vi "UE9 Pin Configuration.vi"(4 "Enable Counter1":bool, 6 "Enable Counter0":bool, 8 "error in":errorcluster, 9 "Enable DACs":bool, 10 "Number of Timers Enabled":u8, 11 "Handle In":i32) -> (0 "error out":errorcluster, 3 "Handle Out":i32)   [LabVIEW 2021]
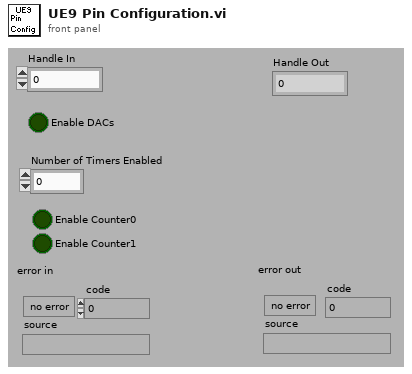
[diagram p1: front panel]
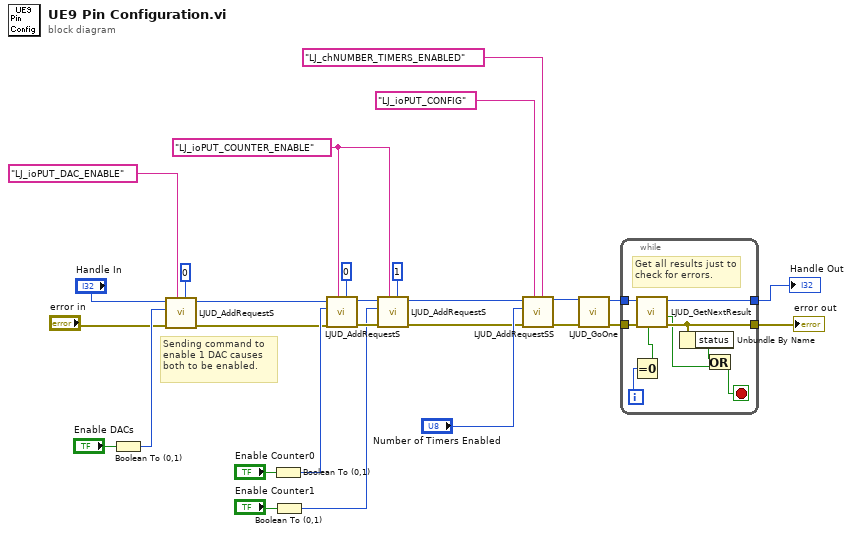
[diagram p0: block diagram]
diagram:
  w19 = "LJ_ioPUT_COUNTER_ENABLE" ("Channel")
  # "Sending command to\nenable 1 DAC causes\nboth to be enabled."
  n1 = Boolean To (0,1)(Boolean="Enable DACs") -> (0, 1=w5:i16)
  n2 = call "LJUD_AddRequestS.vi"("Channel"=0, "IOType"="LJ_ioPUT_DAC_ENABLE" ("Channel"), "error in"="error in", "Value"=w5, "Handle In"="Handle In") -> ("error out"=w9:errorcluster, "Handle Out"=w8:i32)  [unwired: 5 in]
  n3 = Boolean To (0,1)(Boolean="Enable Counter0") -> (0, 1=w13:i16)
  n4 = Boolean To (0,1)(Boolean="Enable Counter1") -> (0, 1=w12:i16)
  n5 = call "LJUD_AddRequestS.vi"("Channel"=0, "IOType"=w19, "error in"=w9, "Value"=w13, "Handle In"=w8) -> ("error out"=w21:errorcluster, "Handle Out"=w20:i32)  [unwired: 5 in]
  n6 = call "LJUD_AddRequestS.vi"("Channel"=1, "IOType"=w19, "error in"=w21, "Value"=w12, "Handle In"=w20) -> ("error out"=w1:errorcluster, "Handle Out"=w2:i32)  [unwired: 5 in]
  n7 = call "LJUD_AddRequestSS.vi"("Channel"="LJ_chNUMBER_TIMERS_ENABLED", "IOType"="LJ_ioPUT_CONFIG", "error in"=w1, "Value"="Number of Timers Enabled", "Handle In"=w2) -> ("error out"=w28:errorcluster, "Handle Out"=w27:i32)  [unwired: 5 in]
  n8 = call "LJUD_GoOne.vi"("error in"=w28, "Handle In"=w27) -> ("error out"=w26:errorcluster, "Handle Out"=w25:i32)  [unwired: 8 in]
  n9 = while {
    tunnel: [w31] -> w14
    tunnel: [w33] -> w22
    tunnel: w25 -> [w34]
    tunnel: w26 -> [w35]
    i -> [w30]
    stop <- w37 stop-if-true
    # "Get all results just to\ncheck for errors."
    n10 = Equal To 0?(x=w30) -> (x = 0?=w36:bool)
    n11 = call "LJUD_GetNextResult.vi"("GetFirst"=w36, "error in"=w35, "Handle In"=w34) -> ("error out"=w33:errorcluster, "LJE_NO_MORE_DATA_AVAILABLE"=w29:bool, "Handle Out"=w31:i32)  [unwired: 3 in, 3 out]
    n12 = Unbundle By Name(w33) -> ("status"=w32:bool)
    n13 = Or(x=w32, y=w29) -> (x .or. y?=w37:bool)
  }
  "error out" <- w22
  "Handle Out" <- w14
